vi "Int to Memory Cell.vi"(10 "Numeric":i32) -> (2 "Memory Cell":T1={"type"=enum."vector", "x"=0.0, "y"=0.0, "z"=0.0, "w"=0.0})   [LabVIEW 2023]
uses:
  Type Definitions/Memory Cell.ctl
  Type Definitions/Memory Cell Type Enum.ctl
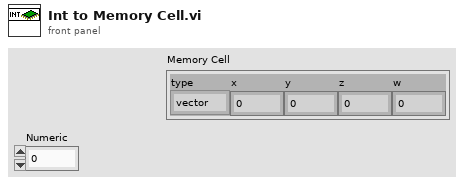
[diagram p1: front panel]
types:
  T1 = typedef "Memory Cell.ctl" = cluster{"type":T2, "x":dbl, "y":dbl, "z":dbl, "w":dbl}
  T2 = typedef "Memory Cell Type Enum.ctl" = enum16{"integer", "float", "vector", "rotation"}
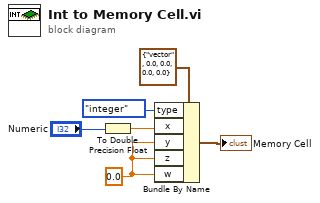
[diagram p0: block diagram]
diagram:
  w1 = 0.0 ("w")
  n1 = To Double Precision Float(number="Numeric") -> (double precision float=w2:dbl)
  n2 = Bundle By Name(cluster=T1 {"type"=enum."vector", "x"=0.0, "y"=0.0, "z"=0.0, "w"=0.0} ("Memory Cell 2"), "type"=Memory_Cell_Type_Enum."integer", "x"=w2, "y"=w1, "z"=w1, "w"=w1) -> (→"Memory Cell":T1)
